vi "SCMP FITS - Define FITS Keywords.vi"() -> (0 "Extension Comments":string[](array[string])=["", "BITS PER PIXEL", "NUMBER OF AXES (2)", "XDIM (PIXELS)", "YDIM (PIXELS)", "4 POLARIZATION STATES", "", "TIME OF OBSERVATION (UTC)", "DATE OF OBSERVATION END (UTC)", "EXPOSURE TIME (MILLISEC)", "", "32768.", "1", "NUMBER OF IMAGES AT EACH STATE", "WAVELENGTH OF OBS (NM)", "", "", "", "", "", "", "", "", "", "", "", "", "", ""], 1 "Extension  Keywords":string[](array[string])=["XTENSION", "BITPIX", "NAXIS", "NAXIS1", "NAXIS2", "NAXIS3", "GCOUNT", "TIME_OBS", "DATE_END", "EXPOSURE", "PCOUNT", "BZERO", "BSCALE", "MODC", "WAVELENG", "COMMENT", "COMMENT", "COMMENT", "COMMENT", "COMMENT", "COMMENT", "COMMENT", "COMMENT", "COMMENT", "COMMENT", "COMMENT", "COMMENT", "COMMENT", "COMMENT"], 2 "Primary Comments":string[](array[string])=["CONFORMS TO FITS STANDARD", "BITS PER PIXEL", "DATA DIMENSIONS IN FITS FILE", "XDIM (PIXELS)", "YDIM (PIXELS)", "4 POLARIZATION STATES", "1 CAMERA", "EXTENSIONS POSSIBLE", "NAME OF OBSERVER", "NAME OF TELESCOPE", "LOCATION OF TELESCOPE", "NAME OF INSTRUMENT", " ADU OFFSET", "CAMERA-STAGE POSITION (MM)", "ROTATIONAL POSITION (DEG)", "0=IN BEAM, 1=OUT OF BEAM", "PRE-FILTER CENTER WAVELENGTH (NM)", "CAL-WHEEL POSITION", "CAMERA SERIAL NUMBER", "FOCAL PLANE TEMP (C)", "LCVR RELAXATION DELAY (mS)", "DATE OF OBSERVATION START (UTC)", "TIME OF OBSERVATION (UTC)", "EXPOSURE TIME (S)", "NUMBER OF IMAGES AT EACH STATE", "TUNING VOLTAGE-1", "TUNING VOLTAGE-2", "TUNING VOLTAGE-3", "TUNING VOLTAGE-4", "TUNING VOLTAGE-5", "BEAM (0=ON BAND OR 1=CONTINUUM)", "WAVELENGTH OF OBS (NM)", "OBSERVER COMMENT", "COOKBOOK  LOADED", "IMAGE TYPE", "SCIENTIFIC GROUP"], 3 "Primary Keywords":string[](array[string])=["SIMPLE", "BITPIX", "NAXIS", "NAXIS1", "NAXIS2", "NAXIS3", "NAXIS4", "EXTEND", "OBSERVER", "TELESCOP", "LOCATION", "INSTRUME", "BZERO", "FOCUS", "ROTPOS", "DIFFUSER", "FW-WVLNG", "FW-CALIB", "CAM-SN1", "CAM-TEMP", "TUNEDLAY", "DATE_OBS", "TIME_OBS", "EXPOSURE", "MODC", "NLC-1", "NLC-2", "NLC-3", "NLC-4", "NLC-5", "BEAM", "WAVELENG", "COMMHEAD", "COOKBOOK", "DATATYPE", "ORIGIN"], 5 "Version":string, 6 "Number of Extension keywords":i32=29, 7 "Number of Primary keywords":i32=36)   [LabVIEW 2014]
uses:
  Controls/Global demo.vi
  <vilib>/Utility/file.llb/Read From Spreadsheet File (string).vi
panel:
  # "Extension Keywords are used for those observational parameters which change on the order\nof the modulation frequency (20 Hz)"
  # "Primay Keywords are used for those instrumental descriptors which change only very\nslowly or not at all during an experiment."
  # "(does not include END)"
  # "36 Keywords will give a header that is a\nmultiple of 2880 if each keyword is 80 characters"
  # "(does not include END)"
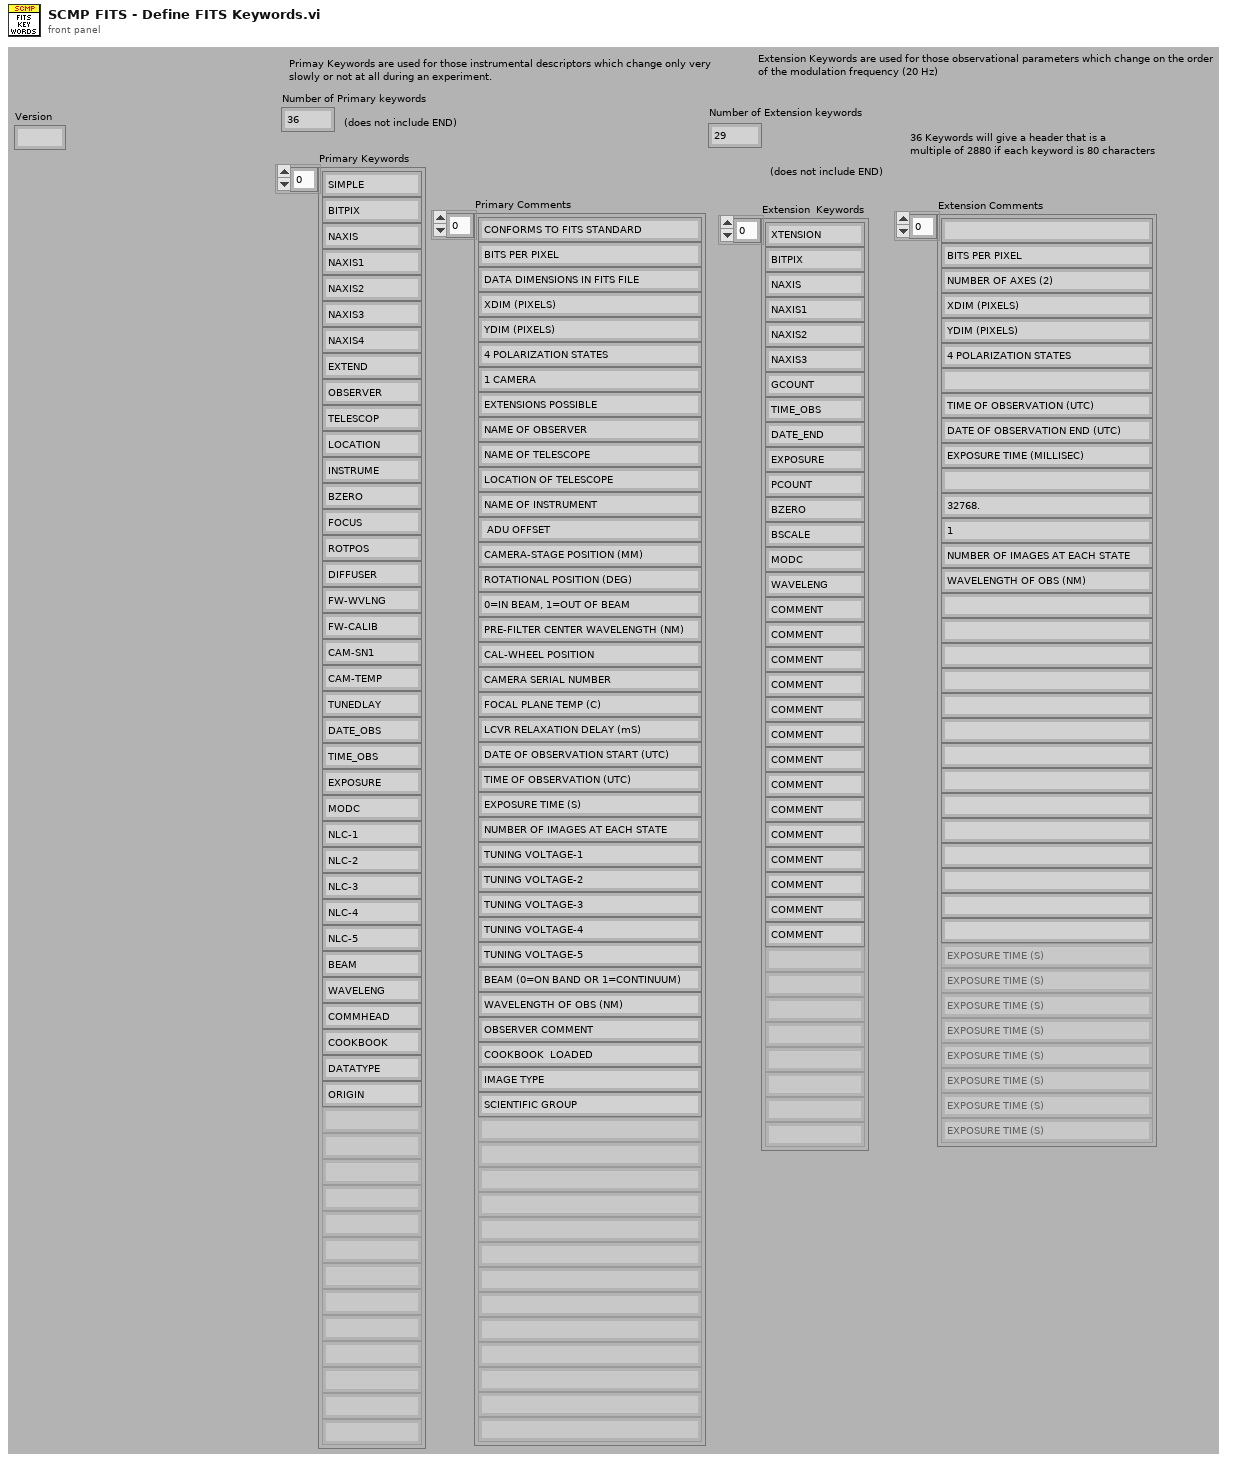
[diagram p1: front panel]
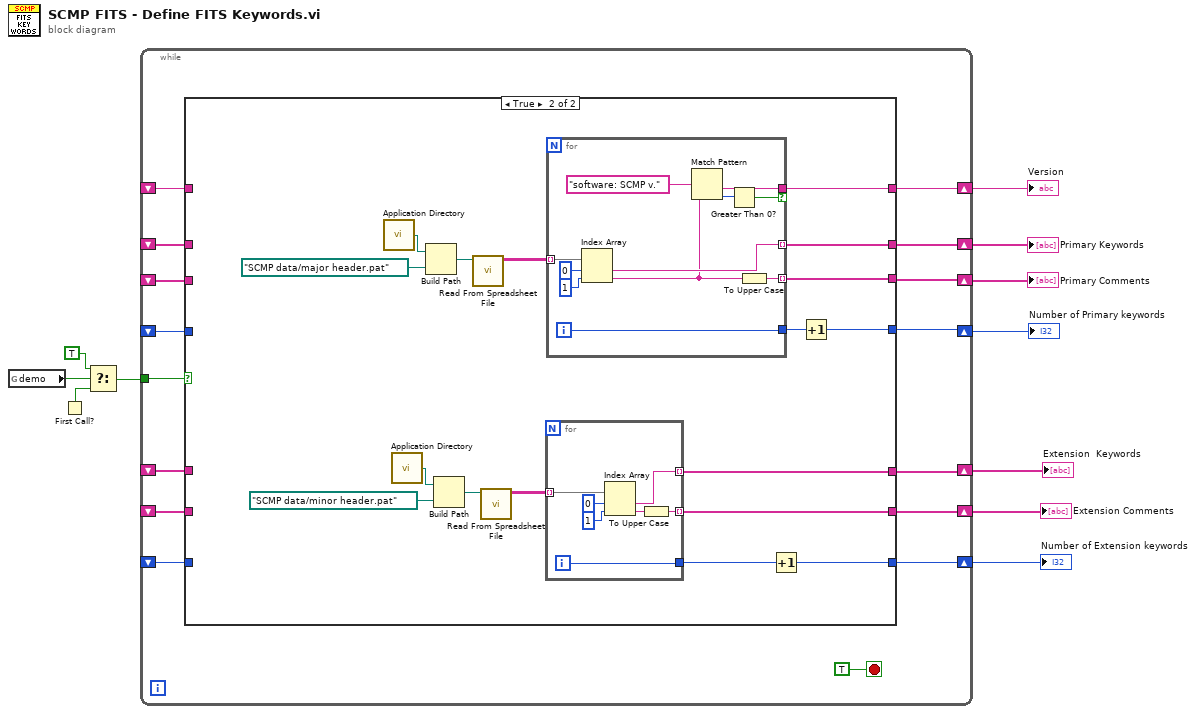
[diagram p0: block diagram]
diagram:
  n1 = global read "Global demo.vi" "demo"() -> (w10:bool)
  n2 = First Call?() -> (First Call?: T/F=w8:bool)
  n3 = Select(t=TRUE ("f"), s=w10, f=w8) -> (s? t:f=w11:bool)
  n4 = while {
    tunnel: w11 -> [w27]
    shift-right: [w25] -> w6
    shift-left: _ -> [w17]
    shift-right: [w24] -> w5
    shift-left: _ -> [w16]
    shift-right: [w23] -> w4
    shift-left: _ -> [w15]
    shift-right: [w22] -> w3
    shift-left: _ -> [w14]
    shift-right: [w21] -> w2
    shift-left: _ -> [w13]
    shift-right: [w20] -> w1
    shift-left: _ -> [w12]
    shift-right: [w19] -> w7
    shift-left: _ -> [w18]
    stop <- TRUE stop-if-true
    n5 = case shown="True" w27 {
      tunnel: [w33 w41] -> w25
      tunnel: [w32 w40] -> w24
      tunnel: [w31 w39] -> w23
      tunnel: [w30 w38] -> w22
      tunnel: [w29 w37] -> w21
      tunnel: [w28 w36] -> w20
      tunnel: [w34 w35] -> w19
      tunnel: w18 -> [w34 _]
      tunnel: w17 -> [w33 _]
      tunnel: w16 -> [w32 _]
      tunnel: w15 -> [w31 _]
      tunnel: w14 -> [w30 _]
      tunnel: w13 -> [w29 _]
      tunnel: w12 -> [w28 _]
      frame False {
      }
      frame True {
        n6 = call <vilib>:"Application Directory.vi"() -> ("Application Directory"=w48:path)
        n7 = call <vilib>:"Application Directory.vi"() -> ("Application Directory"=w44:path)
        n8 = Build Path(base path=w48, name or relative path=path "SCMP data/major header.pat" ("default name")) -> (appended path=w47:path)
        n9 = Build Path(base path=w44, name or relative path=path "SCMP data/minor header.pat" ("default name")) -> (appended path=w43:path)
        n10 = call-poly <vilib>:"Read From Spreadsheet File.vi"("file path (dialog if empty)"=w47) -> ("all rows"=w50:string[][])  [unwired: 6 in, 4 out]
        n11 = call-poly <vilib>:"Read From Spreadsheet File.vi"("file path (dialog if empty)"=w43) -> ("all rows"=w42:string[][])  [unwired: 6 in, 4 out]
        n12 = for {
          tunnel: w42 -> [w58] mode=indexing
          tunnel: [w55] -> w38 mode=indexing
          tunnel: [w52] -> w37 mode=indexing
          tunnel: [w53] -> w46
          i -> [w53]
          n13 = Index Array(array=w58, index #1=0 ("index"), index #2=1 ("index")) -> (element #1=w55:string, element #2=w54:string)
          n14 = To Upper Case(1:w54) -> (0:w52:string)
        }
        n15 = for {
          tunnel: w50 -> [w69] mode=indexing
          tunnel: [w66] -> w41 mode=indexing
          tunnel: [w64] -> w40 mode=indexing
          tunnel: [w65] -> w51
          tunnel: [w60] -> w35 if=w59
          i -> [w65]
          n16 = Index Array(array=w69, index #1=0 ("index"), index #2=1 ("index")) -> (element #1=w66:string, element #2=w62:string)
          n17 = Match Pattern(string=w62, regular expression="software: SCMP v.") -> (after substring=w60:string, offset past match=w61:i32)  [unwired: 1 in, 2 out]
          n18 = Greater Than 0?(x=w61) -> (x > 0?=w59:bool)
          n19 = To Upper Case(1:w62) -> (0:w64:string)
        }
        n20 = Increment(x=w46) -> (x+1=w36:i32)
        n21 = Increment(x=w51) -> (x+1=w39:i32)
      }
    }
  }
  "Primary Keywords" <- w6
  "Primary Comments" <- w5
  "Number of Primary keywords" <- w4
  "Extension Comments" <- w2
  "Extension  Keywords" <- w3
  "Number of Extension keywords" <- w1
  "Version" <- w7
